vi "getWavelength_v80AM3.vi"() -> ()   [LabVIEW 2016]
uses:
  <vilib>/Analysis/baseanly.llb/Mean (DBL).vi
  x32/CLDevIFace.dll
  <vilib>/Analysis/NI_AALBase.lvlib
panel:
  in  "Avg":i32=1
  out "Delta MHz":dbl
  in  "Scale Factor":dbl=800.0
  out "Power (mW)":dbl format="%.9f"
  out "return type":i32
  in  "Clear Chart?":bool
  in  "Delay Time (s)":dbl=0.01
  out "XY Graph":cluster{i32[], dbl[]}(graph)
  out "error out":errorcluster
  out "output param":i32
  in  "stop":bool
  in  "OK Button":bool
  out "Wavelength":dbl format="%.9f"
  in  "CommPort":dbl=5.0 caption="Comm Port #"
  # "Super cavity FSR  6 GHz\nZerodure FSR  750 MHz"
  # "1 pm = 200 MHz @1212nm\n1 pm = 800 MHz @606 nm"
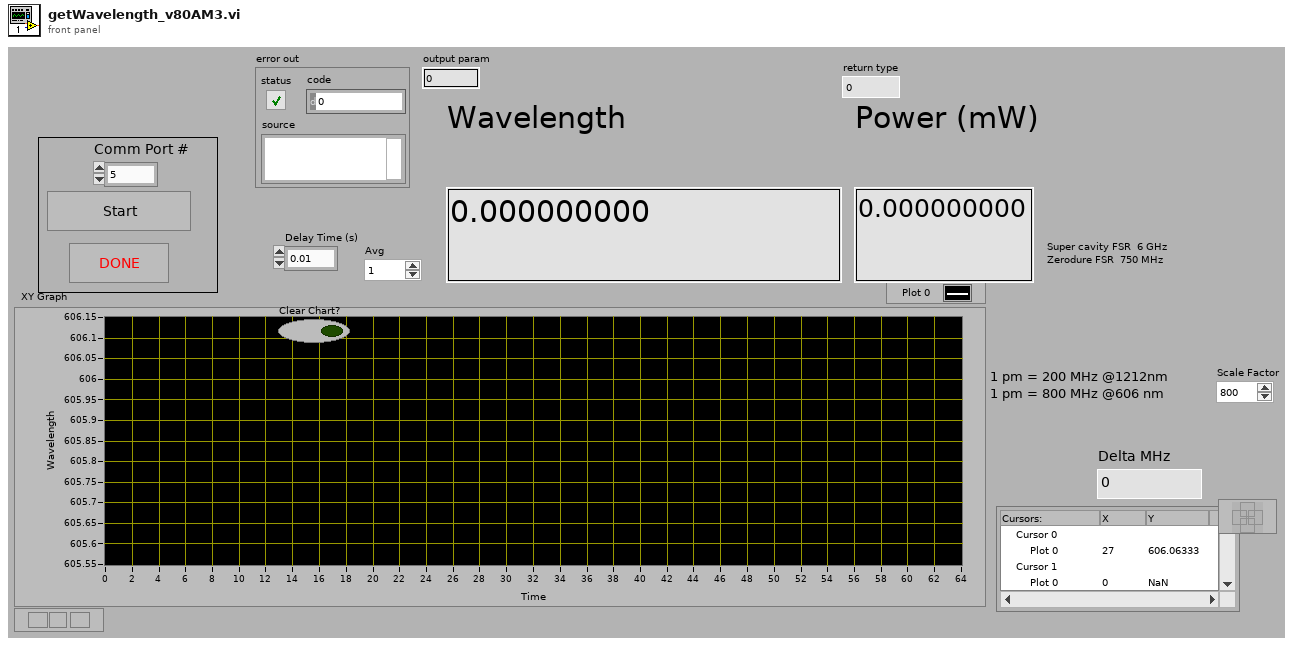
[diagram p1: front panel]
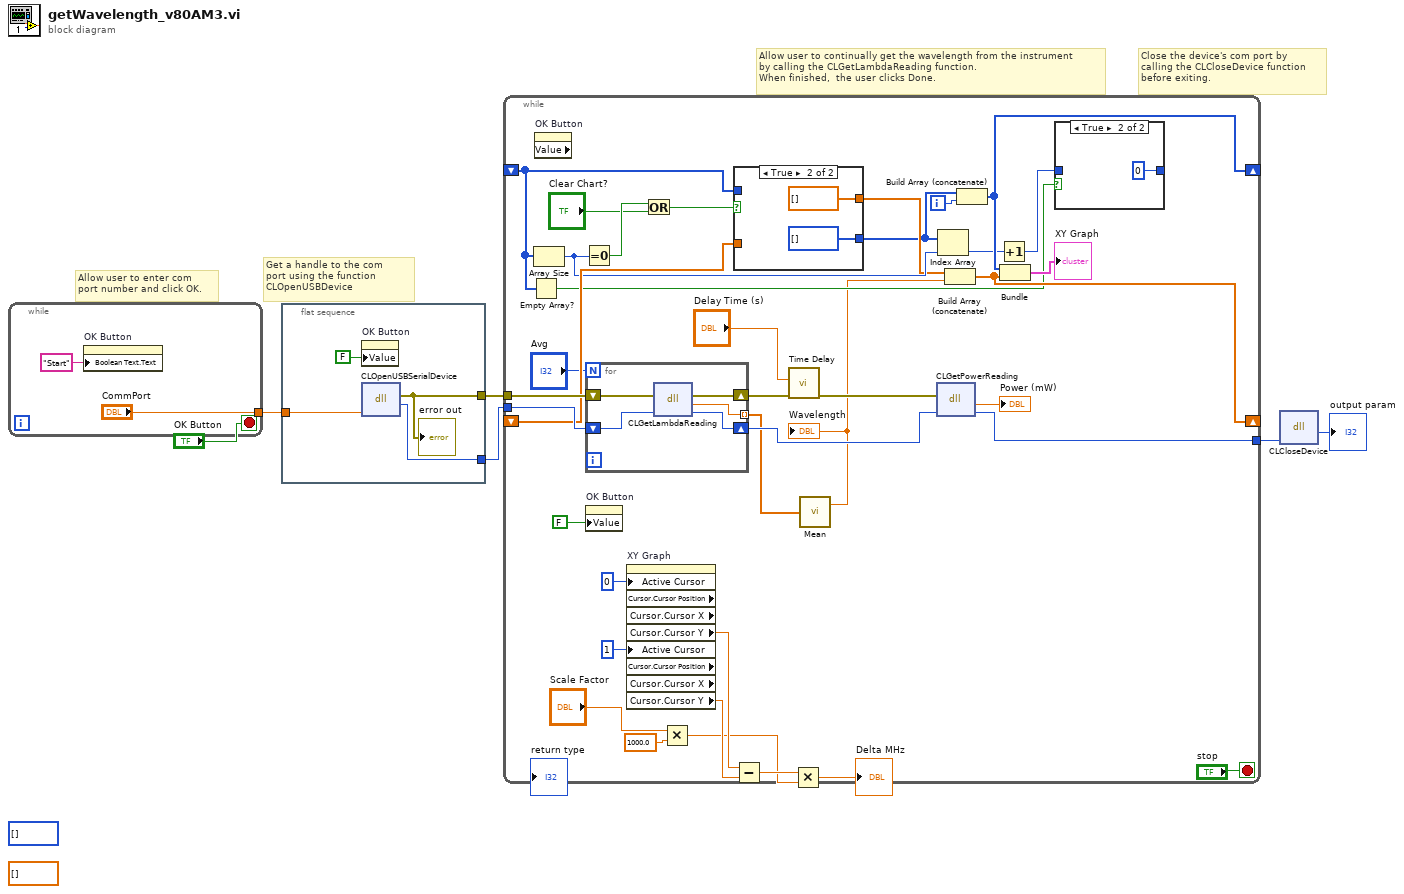
[diagram p0: block diagram]
diagram:
  (unwired) i32[] []
  (unwired) dbl[] []
  # "Close the device's com port by\ncalling the CLCloseDevice function\nbefore exiting."
  # "Allow user to continually get the wavelength from the instrument\nby calling the CLGetLambdaReading function.  \nWhen finished,  the user clicks Done."
  # "Get a handle to the com\nport using the function CLOpenUSBDevice"
  # "Allow user to enter com \nport number and click OK."
  n1 = while {
    tunnel: ["CommPort"] -> w5
    stop <- "OK Button" stop-if-true
    n2 = property on="OK Button" class="Bool (strict)"("Boolean Text.Text"="Start") -> ()  [unwired: 2 in, 2 out]
  }
  n3 = flat-sequence {
    tunnel: w5 -> [w12]
    tunnel: [w11] -> w4
    tunnel: [w9] -> w1
    frame #0 {
      n4 = property on="OK Button" class="Bool (strict)"("Value"=FALSE) -> ()  [unwired: 2 in, 2 out]
      n5 = dll-call lib="C:/Users/Lab/Desktop/Bristol wavemeter 621/00424-2-00 621 customer CD/Programming Interface/x32/CLDevIface.dll" fn="CLOpenUSBSerialDevice"("commPort"=w12) -> (error out=w9:errorcluster, "return type"=w11:i32)  [unwired: 4 in, 1 out]
      "error out" <- w9
    }
  }
  n6 = while {
    tunnel: w4 -> [w49]
    tunnel: [w36] -> w3
    shift-right: [w46] -> _
    shift-left: _ -> [w40]
    shift-right: [w45] -> _
    shift-left: _ -> [w19]
    tunnel: w1 -> [w41]
    i -> [w16]
    stop <- "stop" stop-if-true
    n7 = Empty Array?(array=w19) -> (empty?=w18:bool)
    n8 = Array Size(array=w19) -> (size(s)=w23:i32)
    n9 = property on="OK Button" class="Bool (strict)" props=["Value"]() -> ()  [unwired: 2 in, 3 out]
    n10 = Equal To 0?(x=w23) -> (x = 0?=w26:bool)
    n11 = for {
      N: "Avg" -> [_]
      tunnel: [w53] -> w14 mode=indexing
      shift-right: [w50] -> w37
      shift-left: w49 -> [w54]
      shift-right: [w52] -> w42
      shift-left: w41 -> [w51]
      n12 = dll-call lib="C:/Users/Lab/Desktop/Bristol wavemeter 621/00424-2-00 621 customer CD/Programming Interface/x32/CLDevIface.dll" fn="CLGetLambdaReading"(error in=w51, "devHandle"=w54) -> (error out=w52:errorcluster, "return type"=w53:dbl, "devHandle"=w50:i32)  [unwired: 2 in, 1 out]
    }
    n13 = property on="OK Button" class="Bool (strict)"("Value"=FALSE) -> ()  [unwired: 2 in, 2 out]
    n14 = property on="XY Graph" class="XYGraph (strict)" props=["Active Cursor", "Cursor", "Cursor Position", "Cursor", "Cursor X", "Cursor", "Cursor Y", "Active Cursor", "Cursor", "Cursor Position", "Cursor", "Cursor X", "Cursor", "Cursor Y"]("Active Cursor"=u32 0, "Active Cursor"=u32 1) -> ("Cursor.Cursor Y"=w32:dbl, "Cursor.Cursor Y"=w33:dbl)  [unwired: 2 in, 6 out]
    n15 = Or(x=w26, y="Clear Chart?") -> (x .or. y?=w24:bool)
    n16 = Multiply(x="Scale Factor", y=1000.0) -> (x*y=w27:dbl)
    n17 = case shown="True" w24 {
      tunnel: w40 -> [w58 _]
      tunnel: w19 -> [w57 _]
      tunnel: [w57 i32[] []] -> w21
      tunnel: [w58 dbl[] []] -> w22
      frame False {
      }
      frame True {
      }
    }
    n18 = Subtract(x=w32, y=w33) -> (x-y=w34:dbl)
    n19 = call "Time Delay"("error in (no error)"=w42, "Delay Time (s)"="Delay Time (s)") -> ("error out"=w39:errorcluster)  [unwired: 9 in]
    n20 = Multiply(x=w34, y=w27) -> (x*y=→"Delta MHz":dbl)
    n21 = call-poly <vilib>:"Mean.vi"("X"=w14) -> ("mean"=w13:dbl)  [unwired: 1 out]
    "Wavelength" <- w13
    n22 = dll-call lib="C:/Users/Lab/Desktop/Bristol wavemeter 621/00424-2-00 621 customer CD/Programming Interface/x32/CLDevIface.dll" fn="CLGetPowerReading"(error in=w39, "devHandle"=w37) -> ("return type"=→"Power (mW)":dbl, "devHandle"=w36:i32)  [unwired: 2 in, 2 out]
    n23 = Index Array(array=w21, index=w23) -> (element=w20:i32)
    n24 = Build Array (concatenate)(w22, w13) -> (w46:dbl[])
    n25 = Build Array (concatenate)(w21, w16) -> (w45:i32[])
    n26 = Increment(x=w20) -> (x+1=w17:i32)
    n27 = Bundle(w45, w46) -> (→"XY Graph":cluster{i32[], dbl[]})  [unwired: 1 in]
    n28 = case shown="True" w18 {
      tunnel: w17 -> [w55 _]
      tunnel: [w55 0] -> _
      frame False {
      }
      frame True {
      }
    }
  }
  n29 = dll-call lib="C:/Users/Lab/Desktop/Bristol wavemeter 621/00424-2-00 621 customer CD/Programming Interface/x32/CLDevIface.dll" fn="CLCloseDevice"("commPort"=w3) -> ("return type"=→"output param":i32)  [unwired: 4 in, 2 out]
